vi "EOL Audit Set Switch Output.vi"(4 "Current Data Index In":i32, 5 "Station Index":i32, 6 "Current Data In":sgl[][](array[numeric]), 7 "Express Motion?":bool, 8 "Error In":errorcluster, 9 "task/channels in":refnum<k21> caption="DO Task", 10 "Current Motion":T2, 11 "Switch Output Array":T1[](array[typedef])) -> (0 "Error Out":errorcluster, 2 "Current Data Index Out":i32, 3 "Current Data Out":sgl[][](array[numeric]))   [LabVIEW 2018]
uses:
  02.Type Def's/All Motions.ctl
  02.Type Def's/All Switch Configuration Cluster.ctl
  05.UserVI's/type defs/EOL Global Digital Output Control.ctl
  05.UserVI's/type defs/EOL Global Digital Output Cluster Control.ctl
panel:
  out "Finish?":bool
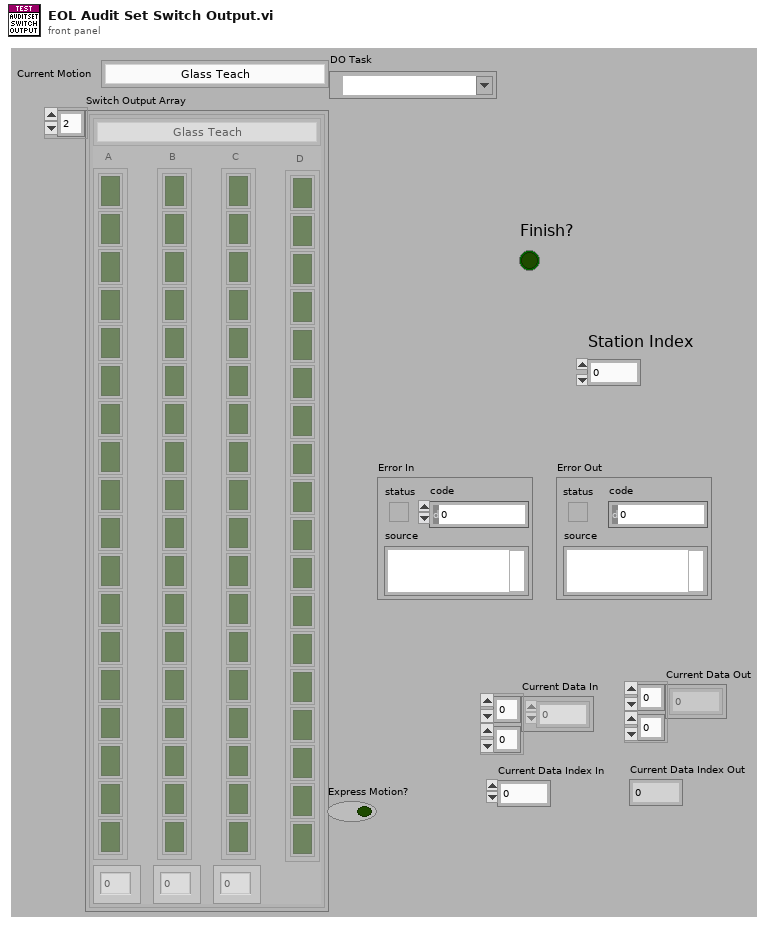
[diagram p1: front panel]
types:
  T1 = typedef "All Switch Configuration Cluster.ctl" = cluster{"All Motions":T2, "A":bool[], "B":bool[], "C":bool[], "D":bool[], "A activation time (ms)":u32, "B activation time (ms)":u32, "C activation time (ms)":u32}
  T2 = typedef "All Motions.ctl" = enum16{"Glass Teach", "Glass Slide Open", "Glass Slide Close", "Glass Vent Open", "Glass Vent Close", "Sunshade Teach", "Sunshade Open", "Sunshade Close", "Idle", "Sunshade Open 2", "Sunshade Close 2", "Glass Slide Open Sunshade Open", "Glass Slide Open Sunshade Close", "Glass Slide Close Sunshade Open", "Glass Slide Close Sunshade Close", "Glass Vent Open Sunshade Open", "Glass Vent Open Sunshade Close", "Glass Vent Close Sunshade Open", "Glass Vent Close Sunshade Close", "Express Glass Slide Open", "Express Glass Slide Close", "Express Glass Vent Open", "Express Glass Vent Close", "Express Sunshade Open", "Express Sunshade Close", "Express Sunshade Open 2", "Express Sunshade Close 2", "Express Glass Slide Open Sunshade Open", "Express Glass Slide Open Sunshade Close", "Express Glass Slide Close Sunshade Open", "Express Glass Slide Close Sunshade Close", "Express Glass Vent Open Sunshade Open", "Express Glass Vent Open Sunshade Close", "Express Glass Vent Close Sunshade Open", "Express Glass Vent Close Sunshade Close", "Goto Position Glass", "Goto Position Sunshade", "Sunshade Teach 2"}
  T3 = typedef "EOL Global Digital Output Control.ctl" = enum16{"Battery", "IGN High", "IGN Low", "LIN", "CAN", "Switch 1", "Switch 2", "Switch 3", "Switch 4", "Switch 5", "Switch 6", "Glass Analog Switch 1", "Glass Analog Switch 2", "Glass Analog Switch 3", "Glass Analog Switch 4", "Sunshade Analog Switch 1", "Sunshade Analog Switch 2", "Sunshade Analog Switch 3", "Sunshade Analog Switch 4", "Glass Motor Relay 1", "Glass Motor Relay 2", "Sunshade Motor Relay 1", "Sunshade Motor Relay 2"}
  T4 = enum16{"Init", "Write", "Write All", "Clear All", "Stop", "Read"}
  T5 = typedef "EOL Global Digital Output Cluster Control.ctl" = cluster{"Status":bool, "Global DO Ch":T3}
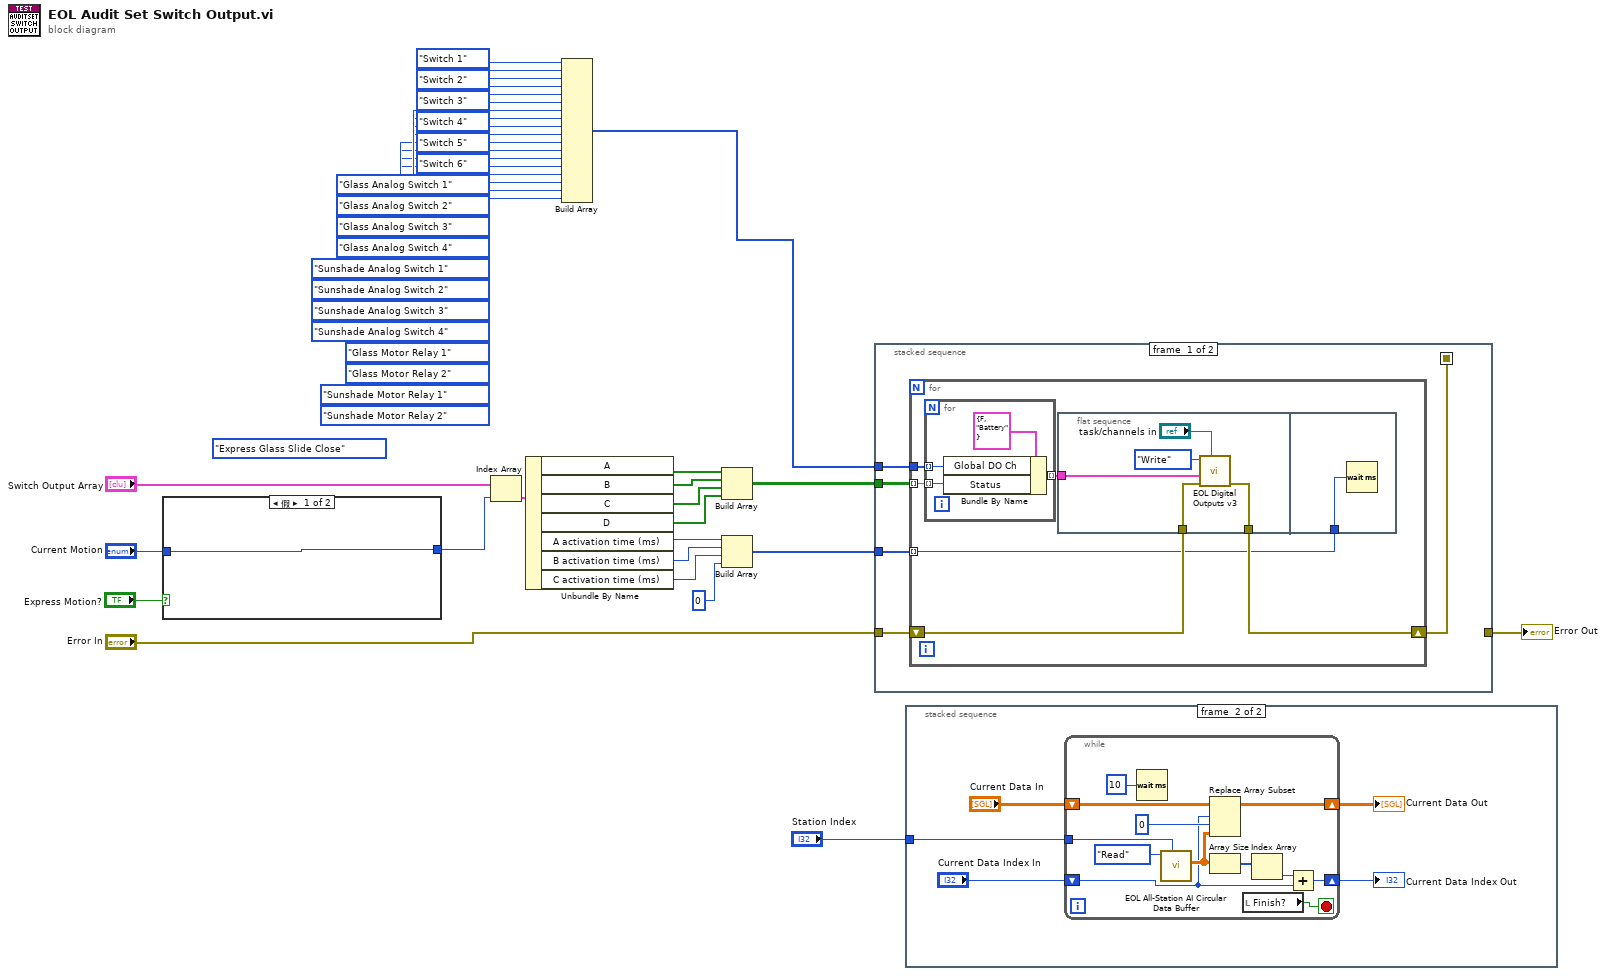
[diagram p0: block diagram]
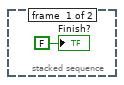
[diagram p2: hidden frame]
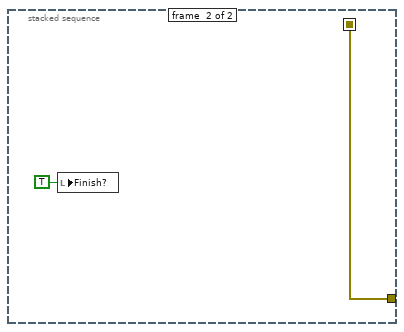
[diagram p3: hidden frame]
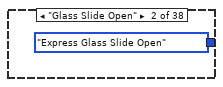
[diagram p6: hidden frame]
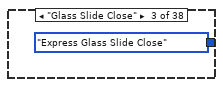
[diagram p7: hidden frame]
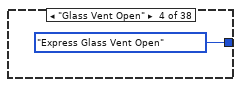
[diagram p8: hidden frame]
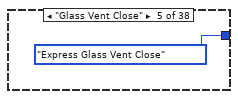
[diagram p9: hidden frame]
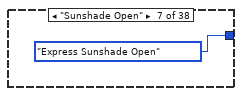
[diagram p11: hidden frame]
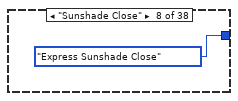
[diagram p12: hidden frame]
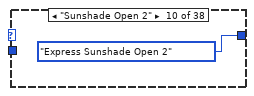
[diagram p14: hidden frame]
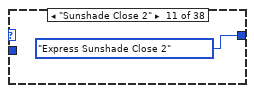
[diagram p15: hidden frame]
diagram:
  (unwired) All_Motions."Express Glass Slide Close" ("Current Motion")
  n1 = case shown="假" "Express Motion?" {
    tunnel: [w38 w40] -> w22
    tunnel: "Current Motion" -> [w38 w39]
    frame False {
    }
    frame True {
      n2 = case shown="\"Sunshade Teach 2\"" w39 {
        selector: w39 -> [_ _ _ _ _ _ _ _ _ _ _ _ _ _ _ _ _ _ _ w60 w61 w62 w63 _ _ _ _ _ _ _ _ _ _ _ _ _ _ _]
        tunnel: [w41 All_Motions."Express Glass Slide Open" ("Current Motion") All_Motions."Express Glass Slide Close" ("Current Motion") All_Motions."Express Glass Vent Open" ("Current Motion") All_Motions."Express Glass Vent Close" ("Current Motion") w46 All_Motions."Express Sunshade Open" ("Current Motion") All_Motions."Express Sunshade Close" ("Current Motion") w49 All_Motions."Express Sunshade Open 2" ("Current Motion") All_Motions."Express Sunshade Close 2" ("Current Motion") w52 w53 w54 w55 w56 w57 w58 w59 w60 w61 w62 w63 w64 w65 w66 w67 w68 w69 w70 w71 w72 w73 w74 w75 w76 w77 w78] -> w40
        tunnel: w39 -> [w41 _ _ _ _ w46 _ _ w49 _ _ w52 w53 w54 w55 w56 w57 w58 w59 _ _ _ _ w64 w65 w66 w67 w68 w69 w70 w71 w72 w73 w74 w75 w76 w77 w78]
        frame "Glass Teach", Default {
        }
        frame "Glass Slide Open" {
        }
        frame "Glass Slide Close" {
        }
        frame "Glass Vent Open" {
        }
        frame "Glass Vent Close" {
        }
        frame "Sunshade Teach" {
        }
        frame "Sunshade Open" {
        }
        frame "Sunshade Close" {
        }
        frame "Idle" {
        }
        frame "Sunshade Open 2" {
        }
        frame "Sunshade Close 2" {
        }
        frame "Glass Slide Open Sunshade Open" {
        }
        frame "Glass Slide Open Sunshade Close" {
        }
        frame "Glass Slide Close Sunshade Open" {
        }
        frame "Glass Slide Close Sunshade Close" {
        }
        frame "Glass Vent Open Sunshade Open" {
        }
        frame "Glass Vent Open Sunshade Close" {
        }
        frame "Glass Vent Close Sunshade Open" {
        }
        frame "Glass Vent Close Sunshade Close" {
        }
        frame "Express Glass Slide Open" {
        }
        frame "Express Glass Slide Close" {
        }
        frame "Express Glass Vent Open" {
        }
        frame "Express Glass Vent Close" {
        }
        frame "Express Sunshade Open" {
        }
        frame "Express Sunshade Close" {
        }
        frame "Express Sunshade Open 2" {
        }
        frame "Express Sunshade Close 2" {
        }
        frame "Express Glass Slide Open Sunshade Open" {
        }
        frame "Express Glass Slide Open Sunshade Close" {
        }
        frame "Express Glass Slide Close Sunshade Open" {
        }
        frame "Express Glass Slide Close Sunshade Close" {
        }
        frame "Express Glass Vent Open Sunshade Open" {
        }
        frame "Express Glass Vent Open Sunshade Close" {
        }
        frame "Express Glass Vent Close Sunshade Open" {
        }
        frame "Express Glass Vent Close Sunshade Close" {
        }
        frame "Goto Position Glass" {
        }
        frame "Goto Position Sunshade" {
        }
        frame "Sunshade Teach 2" {
        }
      }
    }
  }
  n3 = Index Array(array="Switch Output Array", index=w22) -> (element=w36:T1)
  n4 = Unbundle By Name(w36) -> ("A"=w35:bool[], "B"=w34:bool[], "C"=w33:bool[], "D"=w32:bool[], "A activation time (ms)"=w28:u32, "B activation time (ms)"=w27:u32, "C activation time (ms)"=w26:u32)
  n5 = Build Array(EOL_Global_Digital_Output_Control."Switch 1" ("Global DO Ch"), EOL_Global_Digital_Output_Control."Switch 2" ("Global DO Ch"), EOL_Global_Digital_Output_Control."Switch 3" ("Global DO Ch"), EOL_Global_Digital_Output_Control."Switch 4" ("Global DO Ch"), EOL_Global_Digital_Output_Control."Switch 5" ("Global DO Ch"), EOL_Global_Digital_Output_Control."Switch 6" ("Global DO Ch"), EOL_Global_Digital_Output_Control."Glass Analog Switch 1" ("Global DO Ch"), EOL_Global_Digital_Output_Control."Glass Analog Switch 2" ("Global DO Ch"), EOL_Global_Digital_Output_Control."Glass Analog Switch 3" ("Global DO Ch"), EOL_Global_Digital_Output_Control."Glass Analog Switch 4" ("Global DO Ch"), EOL_Global_Digital_Output_Control."Sunshade Analog Switch 1" ("Global DO Ch"), EOL_Global_Digital_Output_Control."Sunshade Analog Switch 2" ("Global DO Ch"), EOL_Global_Digital_Output_Control."Sunshade Analog Switch 3" ("Global DO Ch"), EOL_Global_Digital_Output_Control."Sunshade Analog Switch 4" ("Global DO Ch"), EOL_Global_Digital_Output_Control."Glass Motor Relay 1" ("Global DO Ch"), EOL_Global_Digital_Output_Control."Glass Motor Relay 2" ("Global DO Ch"), EOL_Global_Digital_Output_Control."Sunshade Motor Relay 1" ("Global DO Ch"), EOL_Global_Digital_Output_Control."Sunshade Motor Relay 2" ("Global DO Ch")) -> (w1:T3[])
  n6 = Build Array(w35, w34, w33, w32) -> (w31:bool[][])
  n7 = Build Array(w28, w27, w26, u32 0 ("element")) -> (w24:u32[])
  n8 = stacked-sequence {
    seq-local: [w79 _] -> [_ w101]
    tunnel: w31 -> [w83 _]
    tunnel: [_ w101] -> w30
    tunnel: "Error In" -> [w82 _]
    tunnel: w1 -> [w81 _]
    tunnel: w24 -> [w80 _]
    frame #0 {
      n9 = for {
        tunnel: w83 -> [w89] mode=indexing
        tunnel: w81 -> [w88]
        shift-right: [w86] -> w79
        shift-left: w82 -> [w85]
        tunnel: w80 -> [w84] mode=indexing
        n10 = for {
          tunnel: w89 -> [w98] mode=indexing
          tunnel: w88 -> [w99] mode=indexing
          tunnel: [w97] -> w87 mode=indexing
          n11 = Bundle By Name(cluster=T5 {"Status"=FALSE, "Global DO Ch"=enum."Battery"} ("Cluster"), "Global DO Ch"=w99, "Status"=w98) -> (w97:T5)
        }
        n12 = flat-sequence {
          tunnel: w87 -> [w94]
          tunnel: w85 -> [w93]
          tunnel: [w92] -> w86
          tunnel: w84 -> [w95]
          frame #0 {
            n13 = call "EOL Digital Outputs v3.vi"("task/channels in"="task/channels in", "Error In"=w93, "DO Status"=w94, "Mode"=T4."Write") -> ("Error Out"=w92:errorcluster)  [unwired: 6 in, 1 out]
          }
          frame #1 {
            n14 = Wait (ms)(milliseconds to wait=w95) -> ()  [unwired: 1 out]
          }
        }
      }
    }
    frame #1 {
      n15 = local write "Finish?"(TRUE ("Finish?")) -> ()
    }
  }
  "Error Out" <- w30
  n16 = stacked-sequence {
    tunnel: "Station Index" -> [_ w103]
    frame #0 {
      "Finish?" <- FALSE ("Finish?")
    }
    frame #1 {
      n17 = while {
        shift-right: [w113] -> w105
        shift-left: "Current Data In" -> [w114]
        shift-right: [w111] -> w104
        shift-left: "Current Data Index In" -> [w112]
        tunnel: w103 -> [w108]
        stop <- w109 stop-if-true
        n18 = Wait (ms)(milliseconds to wait=u32 10) -> ()  [unwired: 1 out]
        n19 = call "EOL All-Station AI Circular Data Buffer.vi"("station idx"=w108, "Mode"=enum16{"Initialize", "Read", "Write"}."Read") -> ("Data Read (Samp-Ro, Ch-Col)"=w115:sgl[][])  [unwired: 9 in]
        n20 = Replace Array Subset(array=w114, new element=w115, index (row)=w112, index (col)=0 ("disabled index (col)")) -> (w113:sgl[][])
        n21 = Array Size(array=w115) -> (size(s)=w119:i32[])
        n22 = local read "Finish?"() -> (w109:bool)
        n23 = Index Array(array=w119) -> (element=w117:i32)  [unwired: 1 in]
        n24 = Add(x=w117, y=w112) -> (x+y=w111:i32)
      }
      "Current Data Index Out" <- w104
      "Current Data Out" <- w105
    }
  }
